vi "time_duration_final_count_min.vi"(0 "BD Count":string[](array[string]), 5 "Intime":string[](array[string]), 7 "OutTime":string[](array[string]), 9 "bd array size":i32, 11 "error in (no error)":errorcluster) -> (4 "last count in min":dbl[][](array[numeric]), 8 "appended array":dbl[](array[numeric]) format="%.0g", 10 "Numeric out":dbl, 15 "error out":errorcluster)   [LabVIEW 2017]
panel:
  out "Array 2":string[](array[string])
  out "sum":dbl
  out "Array 3":dbl[][](array[numeric])
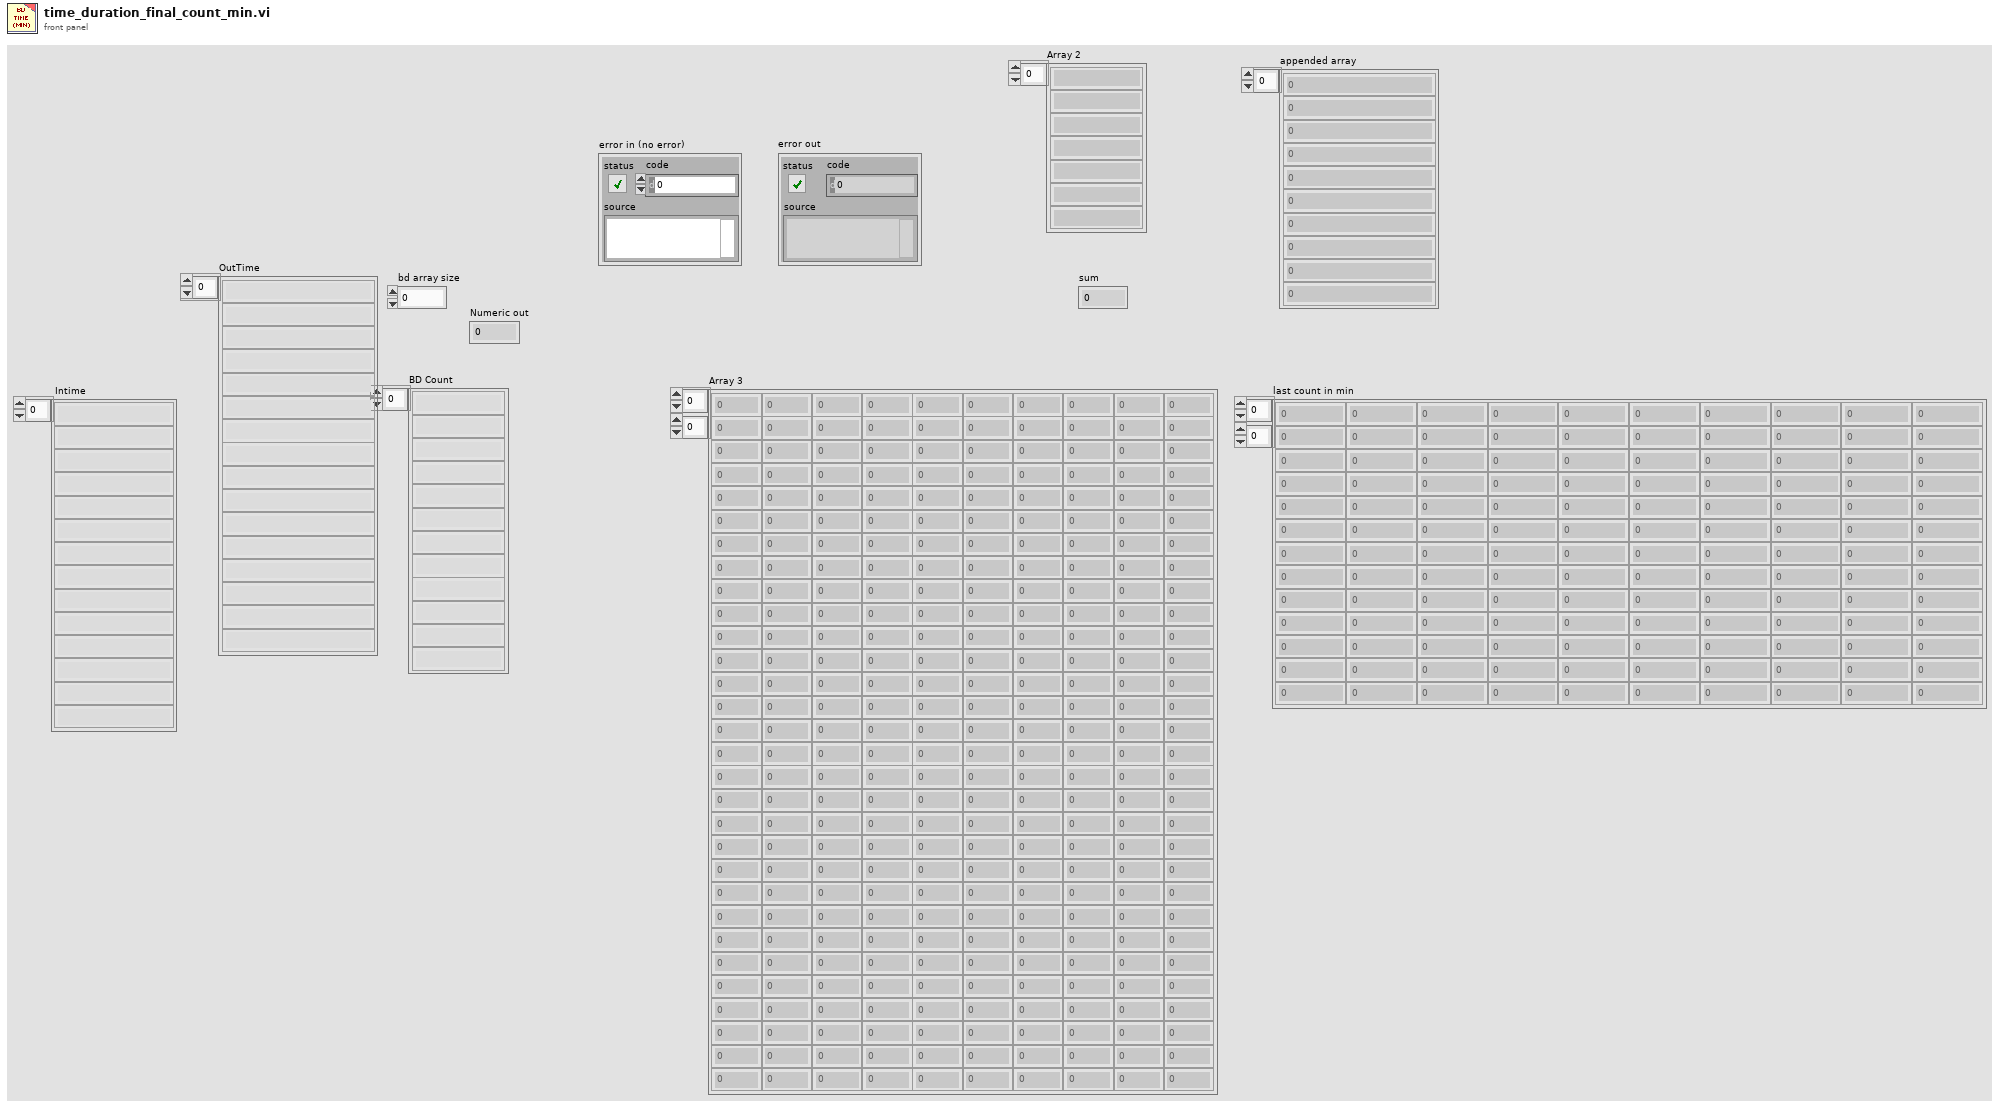
[diagram p1: front panel]
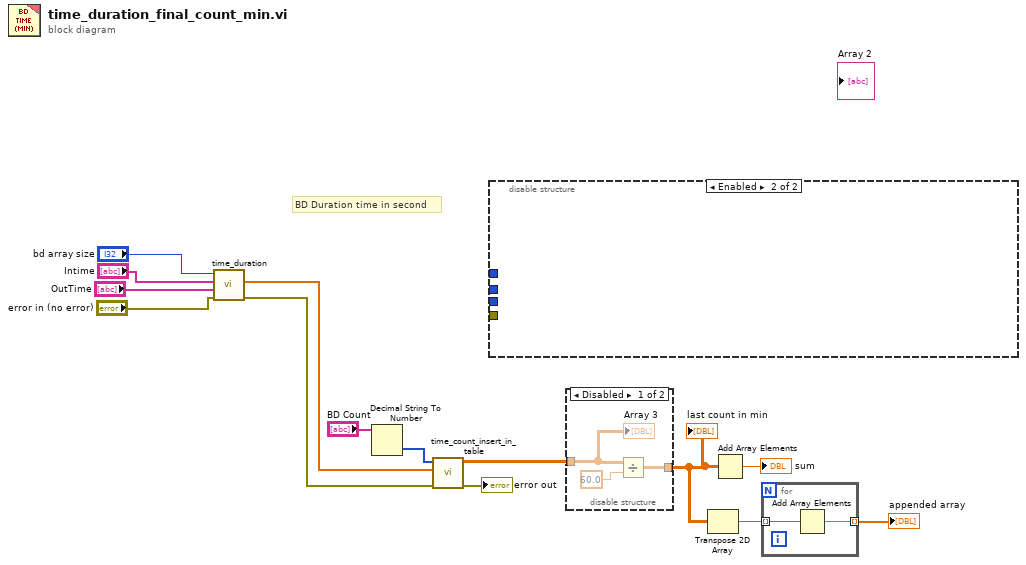
[diagram p0: block diagram]
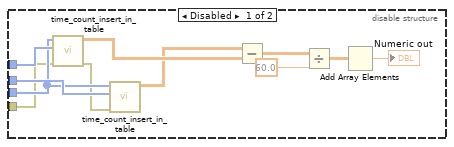
[diagram p3: hidden frame]
diagram:
  # "BD Duration time in second"
  n1 = call "time_duration.vi"("error in (no error)"="error in (no error)", "out time"="OutTime", "in time"="Intime", "Numeric"="bd array size") -> ("error out"=w8:errorcluster, "time in second"=w9:dbl[])  [unwired: 4 in, 2 out]
  n2 = Decimal String To Number(string="BD Count") -> (number=w4:i32[])  [unwired: 2 in, 1 out]
  n3 = call "time_count_insert_in_table.vi"("error in (no error)"=w8, "time in sec"=w9, "bd count array"=w4) -> ("error out"=→"error out":errorcluster, "Array 3"=w7:dbl[][])  [unwired: 7 in]
  n4 = disable-structure shown="Enabled" {
    disable-tunnel: _ -> [w25 _]
    disable-tunnel: _ -> [w24 _]
    disable-tunnel: _ -> [w23 _]
    disable-tunnel: _ -> [w15 _]
    frame Disabled {
      n5 = call "time_count_insert_in_table.vi"("error in (no error)"=w15, "time in sec"=w24, "bd count array"=w23) -> ("error out"=w16:errorcluster, "Array 3"=w18:dbl[][])  [unwired: 7 in]
      n6 = call "time_count_insert_in_table.vi"("error in (no error)"=w16, "time in sec"=w25, "bd count array"=w23) -> ("Array 3"=w17:dbl[][])  [unwired: 7 in, 1 out]
      n7 = Subtract(x=w17, y=w18) -> (x-y=w19:dbl[][])
      n8 = Divide(x=w19, y=60.0) -> (x/y=w21:dbl[][])
      n9 = Add Array Elements(numeric array=w21) -> (sum=→"Numeric out":dbl)
    }
    frame Enabled {
    }
  }
  n10 = disable-structure shown="Disabled" {
    disable-tunnel: w7 -> [w28 w29]
    disable-tunnel: [w26 w29] -> w3
    frame Disabled {
      n11 = Divide(x=w28, y=60.0) -> (x/y=w26:dbl[][])
      "Array 3" <- w28
    }
    frame Enabled {
    }
  }
  "last count in min" <- w3
  n12 = Transpose 2D Array(2D array=w3) -> (transposed array=w2:dbl[][])
  n13 = Add Array Elements(numeric array=w3) -> (sum=→"sum":dbl)
  n14 = for {
    tunnel: w2 -> [w31] mode=indexing
    tunnel: [w30] -> w1 mode=indexing
    n15 = Add Array Elements(numeric array=w31) -> (sum=w30:dbl)
  }
  "appended array" <- w1
